vi "CRYStepSetup Export StepInfo.vi"() -> (0 "pVIRef":refnum<vi>, 1 "sCategory":string, 2 "sStepName":string)   [LabVIEW 2013]
uses:
  CRYStepSetup Global.vi
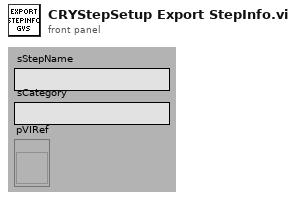
[diagram p1: front panel]
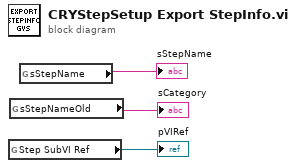
[diagram p0: block diagram]
diagram:
  n1 = global read "CRYStepSetup Global.vi" "Step SubVI Ref"() -> (→"pVIRef":refnum<vi>)
  n2 = global read "CRYStepSetup Global.vi" "sStepNameOld"() -> (→"sCategory":string)
  n3 = global read "CRYStepSetup Global.vi" "sStepName"() -> (→"sStepName":string)
